vi "Create SimpleText Paragraph.vi"(8 "error in (no error)":errorcluster, 10 "simpleText":string, 11 "ooWriter in":refnum<class "ooWriter.lvclass">) -> (0 "error out":errorcluster, 2 "SimpleTextParagraph":refnum<k24>, 3 "ooWriter out":refnum<class "ooWriter.lvclass">)   [LabVIEW 2009, in "ooWriter.lvclass"]
uses:
  ooWriter.lvclass
  C:/Projets/LAVAG/OpenOfficeRGT/AODL/DLLs/AODL.dll
  ooWriter.lvclass/ooWriter.ctl
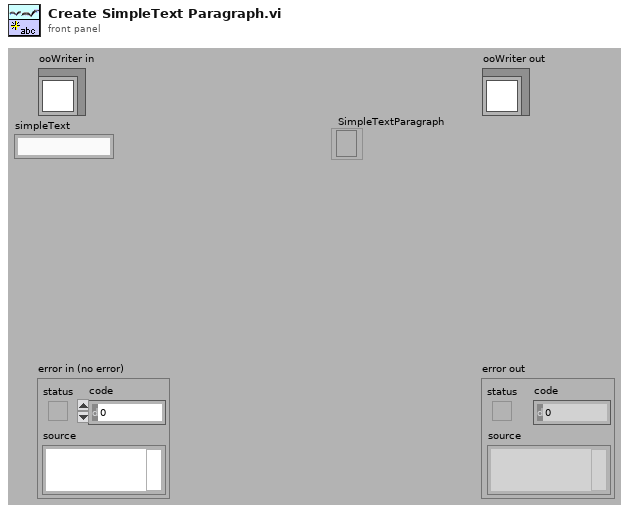
[diagram p1: front panel]
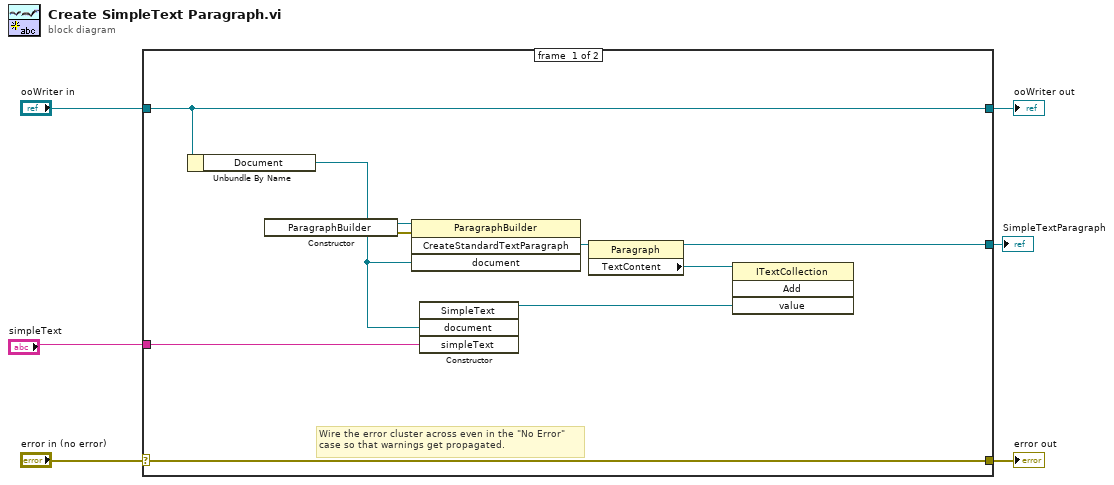
[diagram p0: block diagram]
diagram:
  n1 = case shown="No Error" "error in (no error)" {
    selector: "error in (no error)" -> [w16 w18]
    tunnel: [w16 w18] -> w5
    tunnel: [w10 w17] -> w3
    tunnel: "ooWriter in" -> [w10 w17]
    tunnel: "simpleText" -> [w8 _]
    tunnel: [w7 _] -> w1
    frame #0 {
      # "Wire the error cluster across even in the \"No Error\"\ncase so that warnings get propagated."
      n2 = Unbundle By Name(w10) -> ("Document"=w9:refnum<k24>)
      n3 = constructor class="ParagraphBuilder"() -> (reference out=w14:refnum<k24>, error out=w15:errorcluster)  [unwired: 3 in, 1 out]
      n4 = invoke class="ParagraphBuilder" method="CreateStandardTextParagraph"(reference=w14, error in=w15, "document"=w9) -> ("CreateStandardTextParagraph"=w13:refnum<k24>)  [unwired: 1 in, 3 out]
      n5 = constructor class="SimpleText"("document"=w9, "simpleText"=w8) -> (reference out=w11:refnum<k24>)  [unwired: 3 in, 4 out]
      n6 = property class="Paragraph"(reference=w13) -> (reference out=w7:refnum<k24>, "TextContent"=w12:refnum<k24>)  [unwired: 1 in, 1 out]
      n7 = invoke class="ITextCollection" method="Add"(reference=w12, "value"=w11) -> ()  [unwired: 2 in, 4 out]
    }
    frame #1 {
    }
  }
  "error out" <- w5
  "ooWriter out" <- w3
  "SimpleTextParagraph" <- w1
